vi "Test My Cloneable Module API.vi"() -> ()   [LabVIEW 2025]
doc: "My Module API Tester.\n_____\nBased on DQMH Dev Tools: Project Template 7.1.0.1503."
uses:
  <vilib>/Utility/error.llb/DialogType.ctl
  My Cloneable Module.lvlib
panel:
  out "last error":errorcluster
  in  "Show Diagram on Init":bool
  in  "wait for reply":bool=TRUE
  in  "Run as Singleton?":bool
  in  "Show Block Diagram":bool
  in  "Refresh Modules":bool
  in  "X":dbl=1.0
  out "Reply Payload":dbl
  out "Active Modules":string[](array[string])
  in  "Stop Module":bool
  in  "Select Module":i32(ring)=-1 caption="Select Module\nTo send Request to" items=["All"=-1]
  in  "Run New Module":bool
  out "Do Something Count":i32
  in  "Test Do Something Else and Wait for Reply":bool
  in  "Hide Module Panel":bool
  in  "Show Module Panel":bool
  in  "Test Do Something Else":bool
  in  "Test Do Something":bool
  out "Status":string
  # "This VI tests the API for the Module."
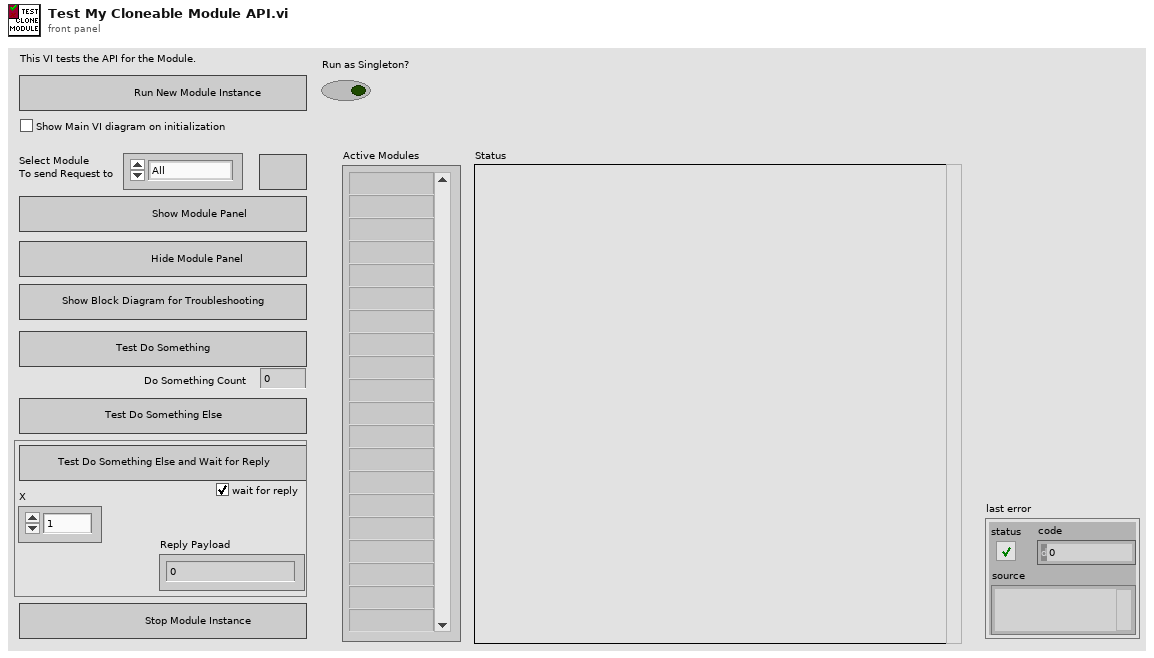
[diagram p1: front panel]
types:
  T1 = typedef "My Cloneable Module.lvlib/Broadcast Events--cluster.ctl" = cluster{"Module Did Init":refnum<user-event>, "Status Updated":refnum<user-event>, "Error Reported":refnum<user-event>, "Did Something":refnum<user-event>, "Module Did Stop":refnum<user-event>, "Update Module Execution Status":refnum<user-event>}
  T2 = typedef "DialogType.ctl" = u16
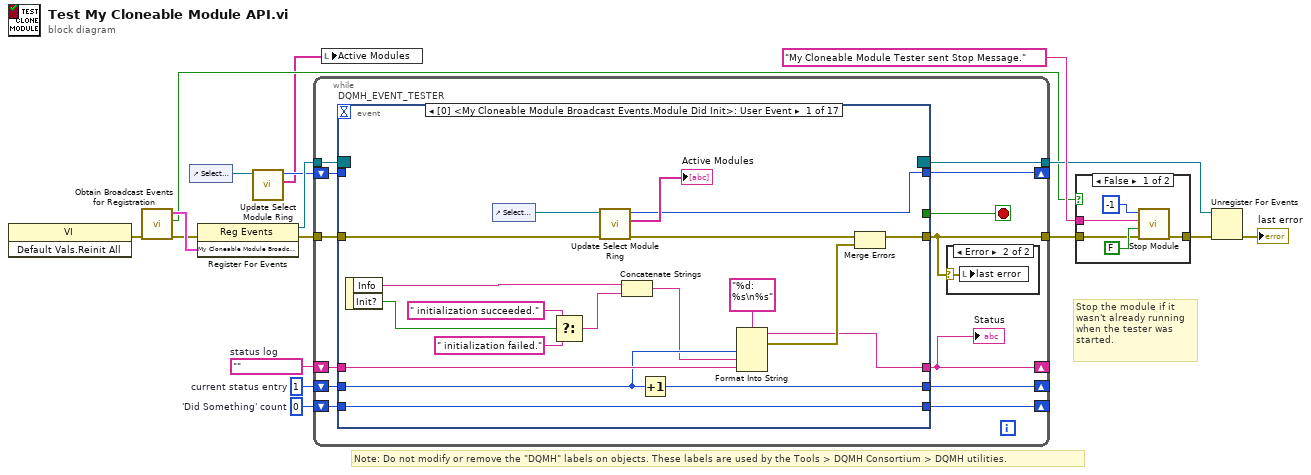
[diagram p0: block diagram]
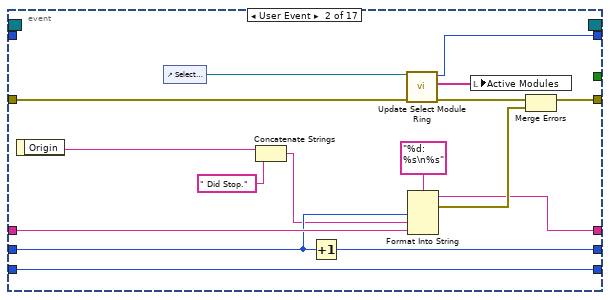
[diagram p4: hidden frame]
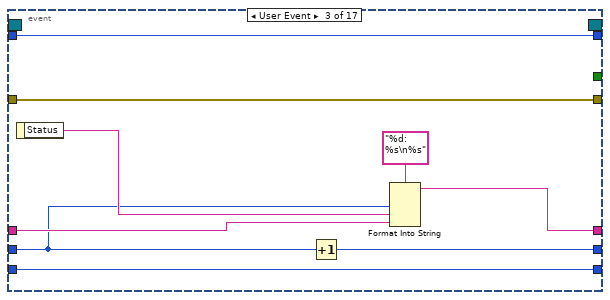
[diagram p5: hidden frame]
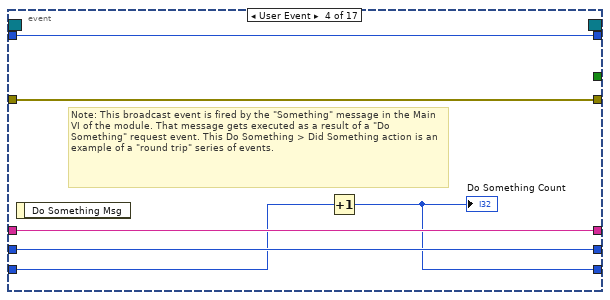
[diagram p6: hidden frame]
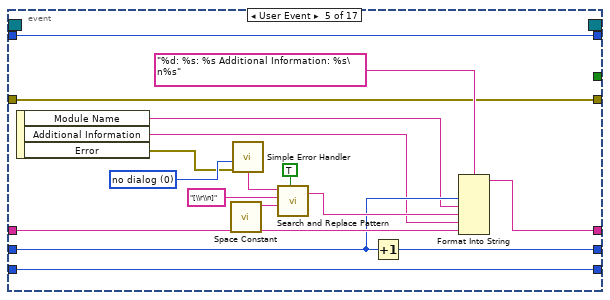
[diagram p7: hidden frame]
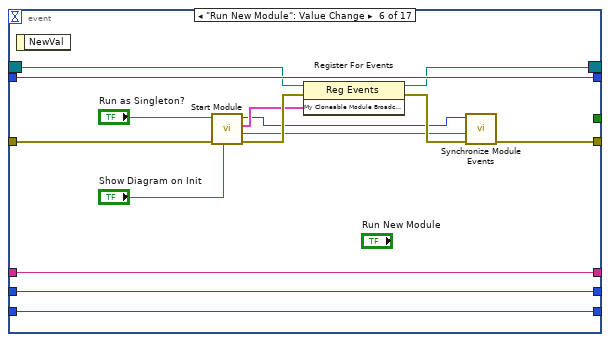
[diagram p8: hidden frame]
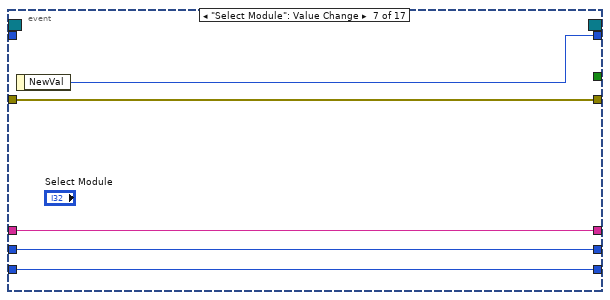
[diagram p9: hidden frame]
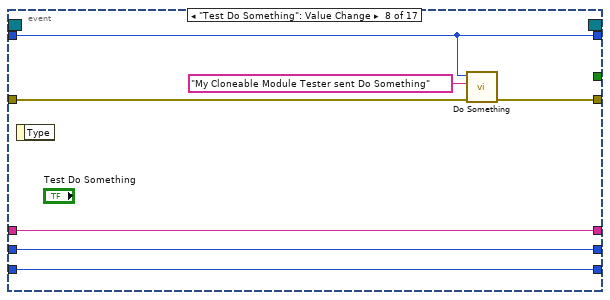
[diagram p10: hidden frame]
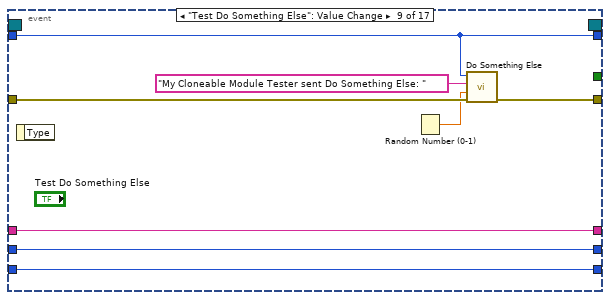
[diagram p11: hidden frame]
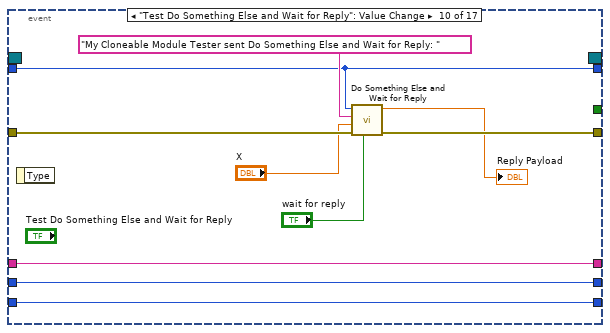
[diagram p12: hidden frame]
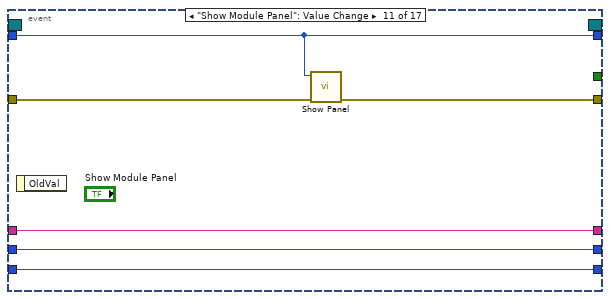
[diagram p13: hidden frame]
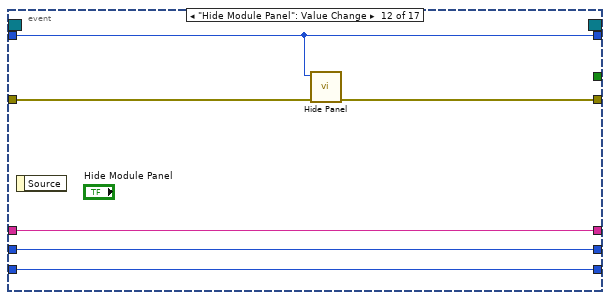
[diagram p14: hidden frame]
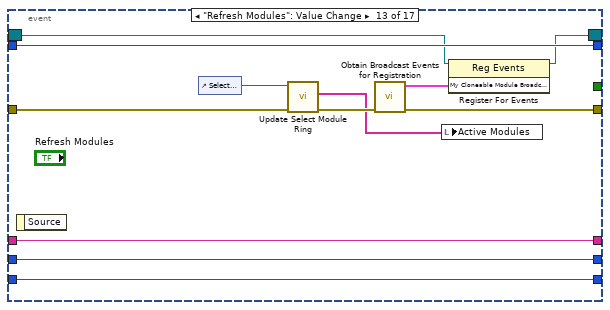
[diagram p15: hidden frame]
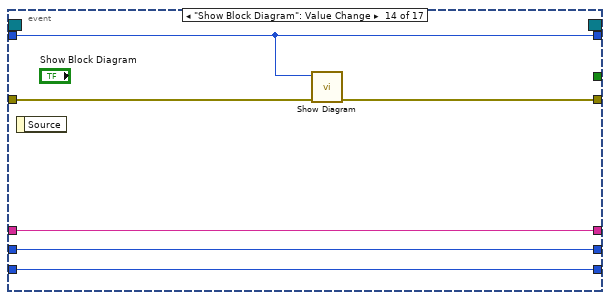
[diagram p16: hidden frame]
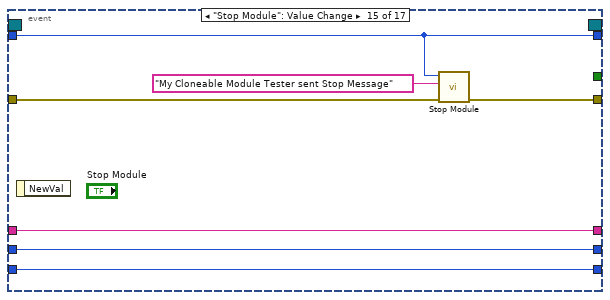
[diagram p17: hidden frame]
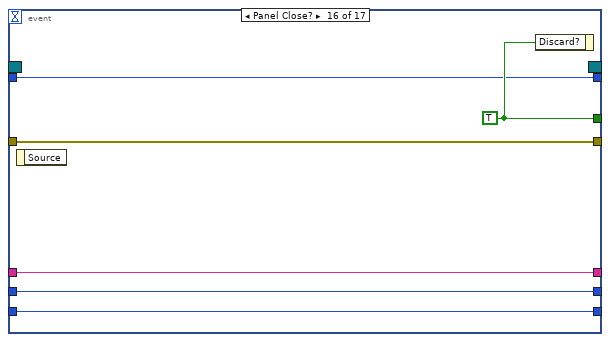
[diagram p18: hidden frame]
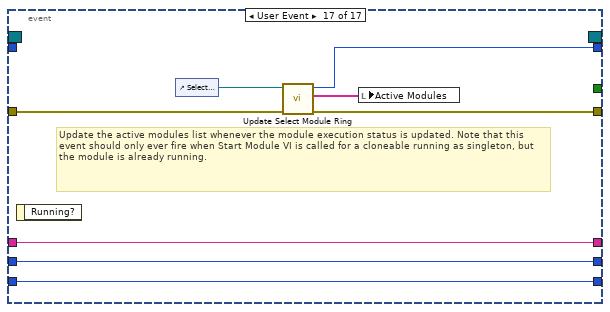
[diagram p19: hidden frame]
diagram:
  w13 = 0  # 'Did Something' count
  w14 = 1  # current status entry
  w15 = ""  # status log
  # "Stop the module if it wasn't already running when the tester was started."
  # "Note: Do not modify or remove the \"DQMH\" labels on objects. These labels are used by the Tools > DQMH Consortium > DQMH utilities."
  n1 = invoke class="VI" method="Default Vals.Reinit All"() -> (error out=w8:errorcluster)  [unwired: 3 in, 2 out]
  n2 = call "Obtain Broadcast Events for Registration.vi"("error in"=w8) -> ("error out"=w7:errorcluster, "Already running?"=w6:bool, "My Cloneable Module Broadcast Events"=w12:T1)  [unwired: 8 in]
  n3 = control-ref of="Select Module"() -> (w3:refnum<vi>)
  n4 = register-events(error in=w7, w12) -> (reference out=w17:refnum<event-registration>, error out=w11:errorcluster)  [unwired: 1 in]
  n5 = call "Update Select Module Ring.vi"("Select Module Ring Ref"=w3) -> ("Active Modules (Array)"=w1:string[], "New Module Ring Value"=w2:i32)  [unwired: 8 in, 1 out]
  n6 = while {
    tunnel: w17 -> [w30]
    tunnel: [w19] -> w5
    tunnel: w11 -> [w29]
    shift-right: [w25] -> _
    shift-left: w15 -> [w27]
    shift-right: [w26] -> _
    shift-left: w14 -> [w28]
    shift-right: [w23] -> _
    shift-left: w13 -> [w24]
    shift-right: [w21] -> _
    shift-left: w2 -> [w22]
    tunnel: [w20] -> w9
    stop <- w18 stop-if-true
    n7 = event "DQMH_EVENT_TESTER" shown="[0] <My Cloneable Module Broadcast Events.Module Did Init>: User Event" {
      selector: w30 -> [_ _ _ _ _ w106 _ _ _ _ _ _ w161 _ _ _ _]
      dyn-events: [_ _ _ _ _ w105 _ _ _ _ _ _ w160 _ _ _ _] -> w20
      timeout: _ -> [_ _ _ _ _ _ _ _ _ _ _ _ _ _ _ _ _]
      tunnel: [_ _ _ _ _ _ _ _ _ _ _ _ _ _ _ w186 _] -> w18
      tunnel: [w39 w57 w75 w81 w85 w104 w118 w124 w132 w143 w148 w154 w157 w169 w175 w185 w189] -> w19
      tunnel: w29 -> [w41 w59 w75 w81 w85 w107 w118 w125 w133 w137 w149 w155 w162 w173 w176 w185 w190]
      tunnel: w28 -> [w47 w63 w67 w79 w88 w110 w116 w121 w128 w140 w146 w152 w166 w171 w179 w183 w193]
      tunnel: w27 -> [w48 w64 w71 w80 w89 w111 w117 w122 w129 w141 w147 w153 w167 w172 w180 w184 w194]
      tunnel: [w45 w61 w72 w80 w87 w111 w117 w122 w129 w141 w147 w153 w167 w172 w180 w184 w194] -> w25
      tunnel: [w46 w62 w74 w79 w86 w110 w116 w121 w128 w140 w146 w152 w166 w171 w179 w183 w193] -> w26
      tunnel: w24 -> [w42 w60 w70 w78 w98 w109 w115 w120 w127 w139 w145 w151 w165 w170 w178 w182 w192]
      tunnel: [w42 w60 w70 w77 w98 w109 w115 w120 w127 w139 w145 w151 w165 w170 w178 w182 w192] -> w23
      tunnel: w22 -> [_ _ w68 w76 w97 w108 _ w119 w126 w138 w144 w150 w164 w168 w177 w181 _]
      tunnel: [w36 w54 w68 w76 w97 w108 w114 w119 w126 w138 w144 w150 w164 w168 w177 w181 w188] -> w21
      event User Event {
        n8 = event-data() -> ("Info"=w44:string, "Init?"=w33:bool)  [unwired: 1 in]
        n9 = control-ref of="Select Module"() -> (w38:refnum<vi>)
        n10 = Select(t=" initialization succeeded.", s=w33, f=" initialization failed.") -> (s? t:f=w32:string)
        n11 = call "Update Select Module Ring.vi"("error in"=w41, "Select Module Ring Ref"=w38) -> ("error out"=w40:errorcluster, "Active Modules (Array)"=→"Active Modules":string[], "New Module Ring Value"=w36:i32)  [unwired: 7 in]
        n12 = Concatenate Strings(w44, w32) -> (w43:string)
        n13 = Increment(x=w47) -> (x+1=w46:i32)
        n14 = Format Into String(format string="%d: %s\n%s", w47, w43, w48) -> (resulting string=w45:string, error out=w50:errorcluster)  [unwired: 2 in]
        n15 = Merge Errors(w40, w50) -> (w39:errorcluster)
      }
      event User Event {
        n16 = event-data() -> ("Origin"=w52:string)  [unwired: 1 in]
        n17 = control-ref of="Select Module"() -> (w56:refnum<vi>)
        n18 = Concatenate Strings(w52, " Did Stop.") -> (w51:string)
        n19 = Increment(x=w63) -> (x+1=w62:i32)
        n20 = call "Update Select Module Ring.vi"("error in"=w59, "Select Module Ring Ref"=w56) -> ("error out"=w58:errorcluster, "Active Modules (Array)"=w55:string[], "New Module Ring Value"=w54:i32)  [unwired: 7 in]
        n21 = Format Into String(format string="%d: %s\n%s", w63, w51, w64) -> (resulting string=w61:string, error out=w66:errorcluster)  [unwired: 2 in]
        n22 = local write "Active Modules"(w55) -> ()
        n23 = Merge Errors(w58, w66) -> (w57:errorcluster)
      }
      event User Event {
        n24 = event-data() -> ("Status"=w69:string)  [unwired: 1 in]
        n25 = Increment(x=w67) -> (x+1=w74:i32)
        n26 = Format Into String(format string="%d: %s\n%s", w67, w69, w71) -> (resulting string=w72:string)  [unwired: 2 in, 1 out]
      }
      event User Event {
        # "Note: This broadcast event is fired by the \"Something\" message in the Main VI of the module. That message gets executed as a result of a \"Do Something\" request event. This Do Something > Did Something action is an example of a \"round trip\" series of events."
        n27 = event-data() -> ()  [unwired: 1 in, 1 out]
        n28 = Increment(x=w78) -> (x+1=w77:i32)
        "Do Something Count" <- w77
      }
      event User Event {
        w90 = T2 0 items=["no dialog", "OK message", "continue or stop message", "OK message + warnings", "continue/stop + warnings"] ("type of dialog (OK msg:1)")
        n29 = event-data() -> ("Module Name"=w84:string, "Additional Information"=w83:string, "Error"=w82:errorcluster)  [unwired: 1 in]
        n30 = call <vilib>:"Space Constant.vi"() -> ("String"=w94:string)
        n31 = call <vilib>:"Simple Error Handler.vi"("type of dialog (OK msg:1)"=w90, "error in (no error)"=w82) -> ("message"=w91:string)  [unwired: 3 in, 4 out]
        n32 = call <vilib>:"Search and Replace Pattern.vi"("string"=w91, "regular expression (\"\")"="[\\r\\n]" ("regular expression (\"\")"), "replace string (\"\")"=w94, "replace all? (F)"=TRUE ("replace all CR/LF with spaces")) -> ("result string"=w92:string)  [unwired: 1 in, 1 out]
        n33 = Increment(x=w88) -> (x+1=w86:i32)
        n34 = Format Into String(format string="%d: %s: %s Additional Information: %s\n%s", w88, w84, w92, w83, w89) -> (resulting string=w87:string)  [unwired: 2 in, 1 out]
      }
      event "Run New Module": Value Change {
        n35 = event-data() -> ()  [unwired: 1 in, 1 out]
        n36 = call "Start Module.vi"("Show Main VI Diagram on Init (F)"="Show Diagram on Init", "error in"=w107, "Run as Singleton? (F)"="Run as Singleton?") -> ("error out"=w112:errorcluster, "Wait for Event Sync?"=w103:bool, "My Cloneable Module Broadcast Events"=w102:T1, "Module ID"=w99:i32)  [unwired: 4 in, 1 out]
        n37 = register-events(reference=w106, error in=w112, w102) -> (reference out=w105:refnum<event-registration>, error out=w113:errorcluster)
        n38 = call "Synchronize Module Events.vi"("error in"=w113, "Wait for Event Sync?"=w103, "Module ID in"=w99) -> ("error out"=w104:errorcluster)  [unwired: 7 in, 1 out]
      }
      event "Select Module": Value Change {
        n39 = event-data() -> ("NewVal"=w114:i32)  [unwired: 1 in]
      }
      event "Test Do Something": Value Change {
        n40 = event-data() -> ()  [unwired: 1 in, 1 out]
        n41 = call "Do Something.vi"("error in"=w125, "Do Something Message"="My Cloneable Module Tester sent Do Something", "Module ID"=w119) -> ("error out"=w124:errorcluster)  [unwired: 8 in]
      }
      event "Test Do Something Else": Value Change {
        n42 = event-data() -> ()  [unwired: 1 in, 1 out]
        n43 = Random Number (0-1)() -> (number: 0 to 1=w130:dbl)
        n44 = call "Do Something Else.vi"("error in"=w133, "X"=w130, "Do Something else Message"="My Cloneable Module Tester sent Do Something Else: " ("Do Something Message"), "Module ID"=w126) -> ("error out"=w132:errorcluster)  [unwired: 7 in]
      }
      event "Test Do Something Else and Wait for Reply": Value Change {
        n45 = event-data() -> ()  [unwired: 1 in, 1 out]
        n46 = call "Do Something Else and Wait for Reply.vi"("wait for reply (T)"="wait for reply", "error in"=w137, "X"="X", "Do Something Else Message"="My Cloneable Module Tester sent Do Something Else and Wait for Reply: " ("Do Something Message"), "Module ID"=w138) -> ("error out"=w143:errorcluster, "Value"=→"Reply Payload":dbl)  [unwired: 4 in, 1 out]
      }
      event "Show Module Panel": Value Change {
        n47 = event-data() -> ()  [unwired: 1 in, 1 out]
        n48 = call "Show Panel.vi"("error in"=w149, "Module ID"=w144) -> ("error out"=w148:errorcluster)  [unwired: 9 in]
      }
      event "Hide Module Panel": Value Change {
        n49 = event-data() -> ()  [unwired: 1 in, 1 out]
        n50 = call "Hide Panel.vi"("error in"=w155, "Module ID"=w150) -> ("error out"=w154:errorcluster)  [unwired: 9 in]
      }
      event "Refresh Modules": Value Change {
        n51 = event-data() -> ()  [unwired: 1 in, 1 out]
        n52 = control-ref of="Select Module"() -> (w163:refnum<vi>)
        n53 = call "Update Select Module Ring.vi"("error in"=w162, "Select Module Ring Ref"=w163) -> ("error out"=w158:errorcluster, "Active Modules (Array)"=w156:string[])  [unwired: 7 in, 1 out]
        n54 = call "Obtain Broadcast Events for Registration.vi"("error in"=w158) -> ("error out"=w157:errorcluster, "My Cloneable Module Broadcast Events"=w159:T1)  [unwired: 8 in, 1 out]
        n55 = local write "Active Modules"(w156) -> ()
        n56 = register-events(reference=w161, w159) -> (reference out=w160:refnum<event-registration>)  [unwired: 1 in, 1 out]
      }
      event "Show Block Diagram": Value Change {
        n57 = event-data() -> ()  [unwired: 1 in, 1 out]
        n58 = call "Show Diagram.vi"("error in"=w173, "Module ID"=w168) -> ("error out"=w169:errorcluster)  [unwired: 9 in]
      }
      event "Stop Module": Value Change {
        n59 = event-data() -> ()  [unwired: 1 in, 1 out]
        n60 = call "Stop Module.vi"("error in"=w176, "Origin"="My Cloneable Module Tester sent Stop Message", "Module ID"=w177) -> ("error out"=w175:errorcluster)  [unwired: 8 in]
      }
      event Panel Close? {
        w186 = TRUE ("Discard?")
        n61 = event-data() -> ()  [unwired: 1 in, 1 out]
        n62 = event-data("Discard?"=w186) -> ()  [unwired: 1 in, 1 out]
      }
      event User Event {
        # "Update the active modules list whenever the module execution status is updated. Note that this event should only ever fire when Start Module VI is called for a cloneable running as singleton, but the module is already running."
        n63 = event-data() -> ()  [unwired: 1 in, 1 out]
        n64 = control-ref of="Select Module"() -> (w191:refnum<vi>)
        n65 = call "Update Select Module Ring.vi"("error in"=w190, "Select Module Ring Ref"=w191) -> ("error out"=w189:errorcluster, "Active Modules (Array)"=w187:string[], "New Module Ring Value"=w188:i32)  [unwired: 7 in]
        n66 = local write "Active Modules"(w187) -> ()
      }
    }
    "Status" <- w25
    n67 = case shown="Error" w19 {
      selector: w19 -> [_ w31]
      frame No Error {
      }
      frame Error {
        n68 = local write "last error"(w31) -> ()
      }
    }
  }
  n69 = local write "Active Modules"(w1) -> ()
  n70 = case shown="False" w6 {
    tunnel: [w199 w200] -> w16
    tunnel: "My Cloneable Module Tester sent Stop Message." ("Origin") -> [w198 _]
    tunnel: w5 -> [w195 w200]
    frame False {
      n71 = call "Stop Module.vi"("error in"=w195, "Wait for Module to stop? (F)"=FALSE ("Wait for Module to stop?"), "Origin"=w198, "Module ID"=-1 ("Stop all")) -> ("error out"=w199:errorcluster)  [unwired: 7 in]
    }
    frame True {
    }
  }
  n72 = Unregister For Events(event registration refnum=w9, error in=w16) -> (error out=→"last error":errorcluster)
